vi "Voltage_to_Thrust.vi"(2 "Right Voltage":dbl step=0.01, 3 "Left Voltage":dbl step=0.01) -> (0 "Right Thrust":dbl, 1 "Left Thrust":dbl)   [LabVIEW 2009]
uses:
  <vilib>/gmath/NI_Gmath.lvlib
panel:
  in  "Right Voltage / Thrust":cluster{"V":dbl, "T":dbl}[](array[cluster])=[{"V"=0.0, "T"=-2.1}, {"V"=0.25, "T"=-2.1}, {"V"=0.5, "T"=-2.07}, {"V"=0.75, "T"=-1.76}, {"V"=1.0, "T"=-1.37}, {"V"=1.25, "T"=-1.05}, {"V"=1.5, "T"=-0.77}, {"V"=1.75, "T"=-0.47}, {"V"=2.0, "T"=-0.23}, {"V"=2.25, "T"=-0.07}, {"V"=2.5, "T"=0.0}, {"V"=2.75, "T"=0.03}, {"V"=3.0, "T"=0.15}, {"V"=3.25, "T"=0.35}, {"V"=3.5, "T"=0.59}, {"V"=3.75, "T"=0.9}, {"V"=4.0, "T"=1.2}, {"V"=4.25, "T"=1.5}, {"V"=4.5, "T"=1.89}, {"V"=4.75, "T"=2.06}, {"V"=5.0, "T"=2.08}]
  in  "Left Voltage / Thrust":cluster{"V":dbl, "T":dbl}[](array[cluster])=[{"V"=0.0, "T"=-2.1}, {"V"=0.25, "T"=-2.1}, {"V"=0.5, "T"=-2.04}, {"V"=0.75, "T"=-1.69}, {"V"=1.0, "T"=-1.35}, {"V"=1.25, "T"=-1.03}, {"V"=1.5, "T"=-0.74}, {"V"=1.75, "T"=-0.45}, {"V"=2.0, "T"=-0.23}, {"V"=2.25, "T"=-0.07}, {"V"=2.5, "T"=0.0}, {"V"=2.75, "T"=0.03}, {"V"=3.0, "T"=0.15}, {"V"=3.25, "T"=0.33}, {"V"=3.5, "T"=0.57}, {"V"=3.75, "T"=0.85}, {"V"=4.0, "T"=1.15}, {"V"=4.25, "T"=1.46}, {"V"=4.5, "T"=1.81}, {"V"=4.75, "T"=1.93}, {"V"=5.0, "T"=1.94}]
  # "Voltage is in V\nThrust in N"
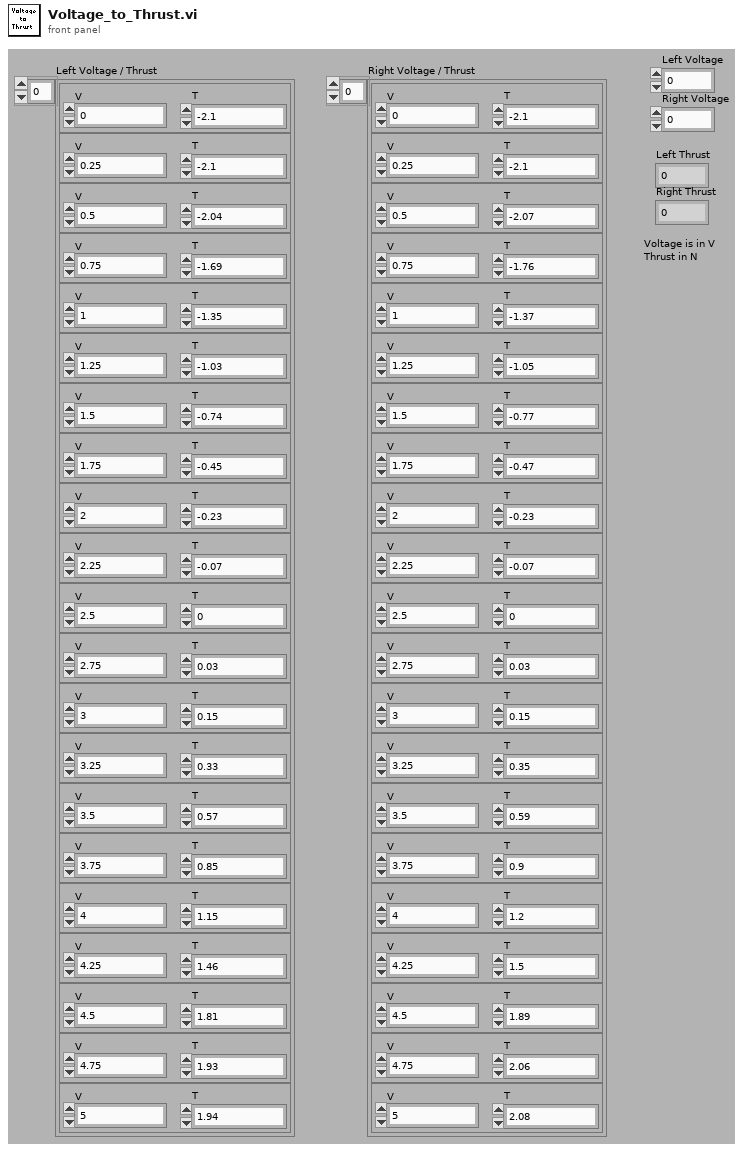
[diagram p1: front panel]
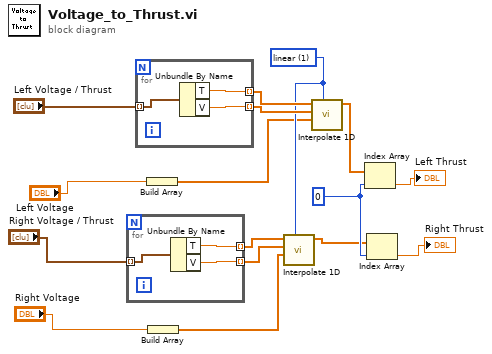
[diagram p0: block diagram]
diagram:
  w5 = 0 ("index")
  w12 = 1 items=["nearest", "linear", "spline", "cubic Hermite", "Lagrange"] ("method")
  n1 = for {
    tunnel: "Right Voltage / Thrust" -> [w19] mode=indexing
    tunnel: [w18] -> w11 mode=indexing
    tunnel: [w17] -> w10 mode=indexing
    n2 = Unbundle By Name(w19) -> ("T"=w18:dbl, "V"=w17:dbl)
  }
  n3 = for {
    tunnel: "Left Voltage / Thrust" -> [w22] mode=indexing
    tunnel: [w21] -> w15 mode=indexing
    tunnel: [w20] -> w14 mode=indexing
    n4 = Unbundle By Name(w22) -> ("T"=w21:dbl, "V"=w20:dbl)
  }
  n5 = Build Array("Left Voltage") -> (w8:dbl[])
  n6 = Build Array("Right Voltage") -> (w6:dbl[])
  n7 = call <vilib>:"Interpolate 1D.vi"("method"=w12, "xi"=w6, "X"=w10, "Y"=w11) -> ("yi"=w1:dbl[])  [unwired: 5 in, 2 out]
  n8 = call <vilib>:"Interpolate 1D.vi"("method"=w12, "xi"=w8, "X"=w14, "Y"=w15) -> ("yi"=w4:dbl[])  [unwired: 5 in, 2 out]
  n9 = Index Array(array=w4, index=w5) -> (element=→"Left Thrust":dbl)
  n10 = Index Array(array=w1, index=w5) -> (element=→"Right Thrust":dbl)
